vi "getPosXY.vi"(8 "Device Y in":refnum<k24>, 10 "Device XY in":T1, 11 "Device X in":refnum<k24>) -> (0 "Device Y out":refnum<k24>, 2 "Device XY out":T2, 3 "Device X out":refnum<k24>)   [LabVIEW 2014]
uses:
  motorsGlobalVar.vi
  C:/user-Lab/AndreTec/GITs/andretec/Thorlabs-Vector-Move/kinesisTec/Kinesis/Thorlabs.MotionControl.TCube.DCServoCLI.dll
  kinesisTec/Kinesis/Thorlabs.MotionControl.TCube.DCServoCLI.dll
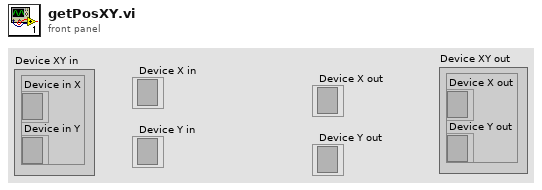
[diagram p1: front panel]
types:
  T1 = cluster{"Device in X":refnum<k24>, "Device in Y":refnum<k24>}
  T2 = cluster{"Device X out":refnum<k24>, "Device Y out":refnum<k24>}
  T3 = cluster{"Device out":refnum<k24>, "Device out":refnum<k24>}
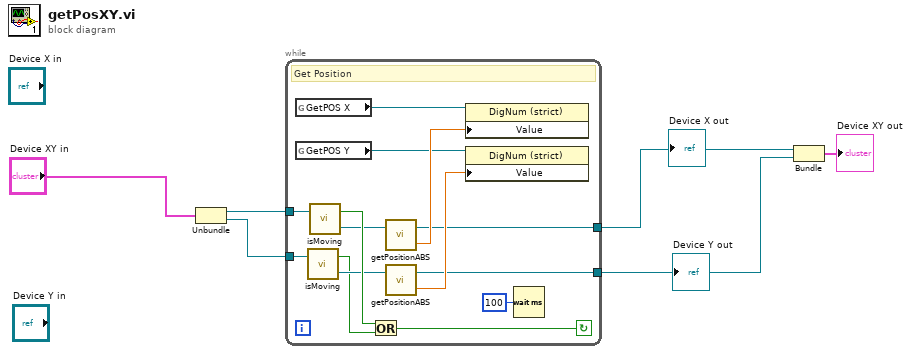
[diagram p0: block diagram]
diagram:
  n1 = Unbundle("Device XY in") -> ("Device in X"=w2:refnum<k24>, "Device in Y"=w3:refnum<k24>)
  n2 = while {
    tunnel: w2 -> [w19]
    tunnel: w3 -> [w20]
    tunnel: [w13] -> w6
    tunnel: [w12] -> w5
    stop <- w15 continue-if-true
    # "Get Position"
    n3 = global read "motorsGlobalVar.vi" "GetPOS X"() -> (w8:refnum<vi>)
    n4 = global read "motorsGlobalVar.vi" "GetPOS Y"() -> (w7:refnum<vi>)
    n5 = call "isMoving.vi"("Device in"=w20) -> ("Device out"=w10:refnum<k24>, "IsMoving"=w9:bool)  [unwired: 1 in]
    n6 = call "isMoving.vi"("Device in"=w19) -> ("Device out"=w11:refnum<k24>, "IsMoving"=w16:bool)  [unwired: 1 in]
    n7 = Or(x=w16, y=w9) -> (x .or. y?=w15:bool)
    n8 = call "getPositionABS.vi"("Device"=w11) -> ("GetPOS"=w18:dbl, "Device out"=w13:refnum<k24>)  [unwired: 1 in]
    n9 = call "getPositionABS.vi"("Device"=w10) -> ("GetPOS"=w17:dbl, "Device out"=w12:refnum<k24>)  [unwired: 1 in]
    n10 = property class="DigNum (strict)"(reference=w8, "Value"=w18) -> ()  [unwired: 1 in, 2 out]
    n11 = property class="DigNum (strict)"(reference=w7, "Value"=w17) -> ()  [unwired: 1 in, 2 out]
    n12 = Wait (ms)(milliseconds to wait=u32 100) -> ()  [unwired: 1 out]
  }
  "Device Y out" <- w5
  "Device X out" <- w6
  n13 = Bundle("Device out"=w6, "Device out"=w5) -> (→"Device XY out":T3)  [unwired: 1 in]
